vi "Configure RF Mixer Maximum Power.vi"(0 "VISA resource name":refnum<visa-resource-name>, 5 "RF Mixer Maximum Power (4 dBm)":dbl=4.0, 11 "error in (no error)":errorcluster) -> (4 "VISA resource name out":refnum<visa-resource-name>, 15 "error out":errorcluster)   [LabVIEW 2014, in "Agilent ESA PSA Series.lvlib"]
doc: "Configures the RF mixer maximum power setting of the Phase Noise personality.\n\n<B>Note:</B>\n\nThis VI is only valid in Phase Noise personality. Use <B>Switch Personality</B> VI to switch to Phase Noise before calling this VI."
uses:
  Agilent ESA PSA Series.lvlib
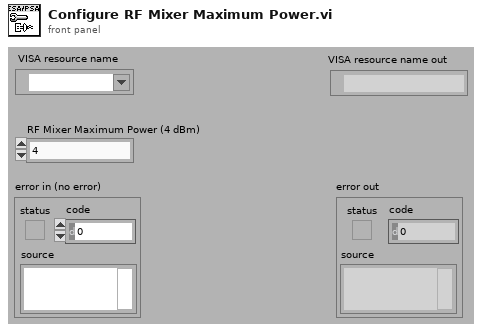
[diagram p1: front panel]
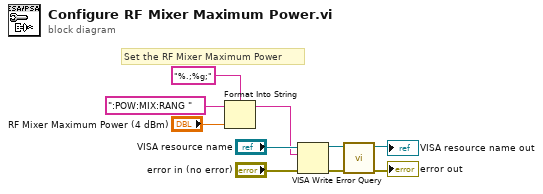
[diagram p0: block diagram]
diagram:
  # "Set the RF Mixer Maximum Power"
  n1 = Format Into String(format string="%.;%g;", initial string=":POW:MIX:RANG ", "RF Mixer Maximum Power (4 dBm)") -> (resulting string=w1:string)  [unwired: 1 in, 1 out]
  n2 = VISA Write(VISA resource name="VISA resource name", write buffer=w1, error in (no error)="error in (no error)") -> (VISA resource name out=w6:refnum<visa-resource-name>, error out=w5:errorcluster)  [unwired: 1 out]
  n3 = call "Error Query.vi"("error in (no error)"=w5, "VISA resource name"=w6) -> ("error out"=→"error out":errorcluster, "VISA resource name out"=→"VISA resource name out":refnum<visa-resource-name>)  [unwired: 6 in, 2 out]
